vi "Step Delay.vi"(8 "error in (no error)":errorcluster, 9 "Step up? (false)":bool, 10 "Channel (T0)":T1 items=["T0", "T1", "A", "B", "C", "D", "E", "F", "G", "H"], 11 "VISA resource name":refnum<visa-resource-name>) -> (0 "error out":errorcluster, 3 "VISA resource name out":refnum<visa-resource-name>, 4 "Device Errors":cluster{"code":i32, "Text":string}[](array[cluster]))   [LabVIEW 2014, in "Stanford Research DG645 - Driver.lvlib"]
doc: "Delay and Output Command: SPDL c,i\nInstrument Error Check\n\nStep delay for channel c by the current step size in the direction i. If i is true, then step up. If i is false, then step down."
uses:
  Stanford Research DG645 - Driver.lvlib
  Channel.ctl
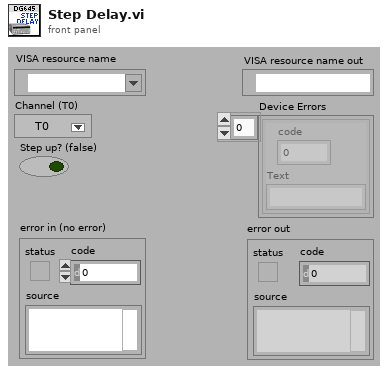
[diagram p1: front panel]
types:
  T1 = typedef "Stanford Research DG645 - Driver.lvlib/Channel.ctl" = i32
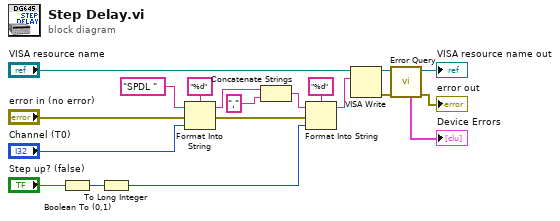
[diagram p0: block diagram]
diagram:
  n1 = Boolean To (0,1)(Boolean="Step up? (false)") -> (0, 1=w4:i16)
  n2 = To Long Integer(number=w4) -> (32bit integer=w1:i32)
  n3 = Format Into String(format string="%d", initial string="SPDL " ("command"), error in="error in (no error)", "Channel (T0)") -> (resulting string=w16:string, error out=w17:errorcluster)
  n4 = Concatenate Strings(w16, "," ("command")) -> (w12:string)
  n5 = Format Into String(format string="%d", initial string=w12, error in=w17, w1) -> (resulting string=w3:string)  [unwired: 1 out]
  n6 = VISA Write(VISA resource name="VISA resource name", write buffer=w3) -> (VISA resource name out=w10:refnum<visa-resource-name>, error out=w7:errorcluster)  [unwired: 1 in, 1 out]
  n7 = call "Error Query.vi"("error in (no error)"=w7, "VISA resource name"=w10) -> ("error out"=→"error out":errorcluster, "VISA resource name out"=→"VISA resource name out":refnum<visa-resource-name>, "Device Errors"=→"Device Errors":cluster{"code":i32, "Text":string}[])  [unwired: 7 in]
